vi "RSZVB Set Pulse Shift Stimulus.vi"(4 "Record Number (1)":i32=1, 5 "Shift Stimulus (0.0 s)":dbl format="%^.3e", 6 "Generator/Port Number (1)":i32=1, 7 "Interface Type (0: Generator)":i32(ring) items=["Generator", "Analyzer Source"], 8 "error in (no error)":errorcluster {"code" format="%.0x"}, 9 "Receiver Type (0: A)":i32(ring) items=["A", "B"], 10 "Channel (1)":i32=1, 11 "VISA session":refnum<visa-resource-name>) -> (0 "error out":errorcluster {"code" format="%.0x"}, 3 "dup VISA session":refnum<visa-resource-name>)   [LabVIEW 2011]
doc: "This VI defines an offset time (shift stimulus) for the wave quantity.\n\nRemote-control command(s):\n[SENSe<Ch>:]PULSe:RECeiver:A<rec_no>:GENerator<gen_no>:TRIGger:DELay <shift_stimulus>\n[SENSe<Ch>:]PULSe:RECeiver:A<rec_no>:SRCPort<port_no>:TRIGger:DELay <shift_stimulus>\n[SENSe<Ch>:]PULSe:RECeiver:B<rec_no>:GENerator<gen_no>:TRIGger:DELay <shift_stimulus>\n[SENSe<Ch>:]PULSe:RECeiver:B<rec_no>:SRCPort<port_no>:TRIGger:DELay <shift_stimulus>"
uses:
  _utility/RSZVB Global Data.vi
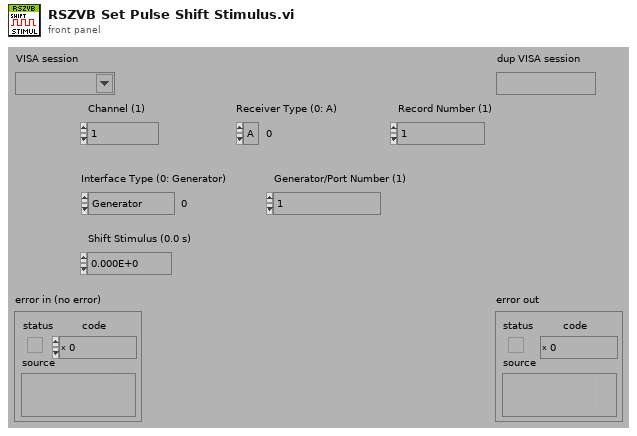
[diagram p1: front panel]
types:
  T1 = cluster{"Error Checking (T: On)":bool, "Installed Options":string[], "Data Valid?":bool, "Ports":i32, "Model":string[], "Option Checking (T: On)":bool}[]
  T2 = cluster{"Error Checking (T: On)":bool, "Installed Options":string[], "Data Valid?":bool, "Ports":i32, "Model":string[], "Option Checking (T: On)":bool}
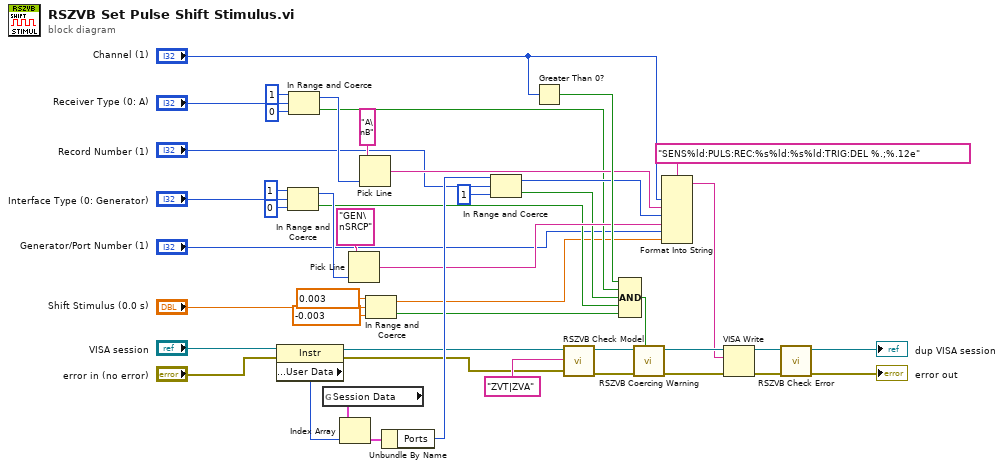
[diagram p0: block diagram]
diagram:
  n1 = property class="Instr"(reference="VISA session", error in="error in (no error)") -> (reference out=w23:refnum<visa-resource-name>, error out=w22:errorcluster, "General Settings:User Data"=w25:u32)
  n2 = In Range and Coerce(upper limit=1, x="Interface Type (0: Generator)", lower limit=0) -> (coerced(x)=w28:i32, In Range?=w15:bool)
  n3 = In Range and Coerce(upper limit=1, x="Receiver Type (0: A)", lower limit=0) -> (coerced(x)=w32:i32, In Range?=w17:bool)
  n4 = global read "RSZVB Global Data.vi" "Session Data"() -> (w26:T1)
  n5 = Index Array(array=w26, index=w25) -> (element=w27:T2)
  n6 = Pick Line(multi-line string="GEN\nSRCP", line index=w28) -> (output string=w18:string)  [unwired: 1 in]
  n7 = Pick Line(multi-line string="A\nB", line index=w32) -> (output string=w20:string)  [unwired: 1 in]
  n8 = In Range and Coerce(upper limit=0.003, x="Shift Stimulus (0.0 s)", lower limit=-0.003) -> (coerced(x)=w13:dbl, In Range?=w14:bool)
  n9 = Unbundle By Name(w27) -> ("Ports"=w24:i32)
  n10 = In Range and Coerce(upper limit=w24, x="Record Number (1)", lower limit=1) -> (coerced(x)=w19:i32, In Range?=w16:bool)
  n11 = Greater Than 0?(x="Channel (1)") -> (x > 0?=w39:bool)
  n12 = call "RSZVB Check Model.vi"("error in (no error)"=w22, "Model"="ZVT|ZVA" ("Options"), "VISA session"=w23) -> ("error out"=w37:errorcluster, "dup VISA session"=w36:refnum<visa-resource-name>)  [unwired: 7 in]
  n13 = Compound Arithmetic op=AND(w39, w17, w16, w15, w14) -> (w41:bool)
  n14 = call "RSZVB Coercing Warning.vi"("In Range?"=w41, "error in (no error)"=w37, "VISA session"=w36) -> ("error out"=w44:errorcluster, "dup VISA session"=w45:refnum<visa-resource-name>)  [unwired: 7 in]
  n15 = Format Into String(format string="SENS%ld:PULS:REC:%s%ld:%s%ld:TRIG:DEL %.;%.12e", "Channel (1)", w20, w19, w18, "Generator/Port Number (1)", w13) -> (resulting string=w40:string)  [unwired: 2 in, 1 out]
  n16 = VISA Write(VISA resource name=w45, write buffer=w40, error in (no error)=w44) -> (VISA resource name out=w42:refnum<visa-resource-name>, error out=w43:errorcluster)  [unwired: 1 out]
  n17 = call "RSZVB Check Error.vi"("error in (no error)"=w43, "VISA session"=w42) -> ("error out"=→"error out":errorcluster, "dup VISA session"=→"dup VISA session":refnum<visa-resource-name>)  [unwired: 8 in]
